vi "filter pipe - plot staff - more - V2.vi"(0 "omega  in":dbl[](array[numeric]), 1 "zin":cdb[](array[numeric]), 2 "z out":cdb[](array[numeric]), 3 "win omega":dbl[](array[numeric]), 4 "phase":dbl[](array[numeric]), 5 "dz/domega in":cdb[](array[numeric]), 6 "center":cdb, 7 "plots: filter related":T6, 8 "norm":dbl, 9 "parameters: complex fit":T1={"main VI path"=path "", "scale factor"=3.0, "# of grid points"=200, "parameters: wavepacket"={"R"=0.5, "wave number"=22.0, "delta k"=7.0, "radii vector"=[], "radial section"=[], "wave vector"=22.0, "wavepacket is"=TRUE}, "span"=0.27789, "interference ?"=enum."cp z center", "filter method"=enum."three"} {"span" min=0.0 max=0.5 step=1e-05 scale=0.0001..0.5 scale format="%#_5f"; "parameters: wavepacket"."delta k" format="%#_3f"; "parameters: wavepacket"."wave number" format="%#_3f"; "parameters: wavepacket"."R" format="%#_3f"}, 11 "tale of three indices -- int -- control":T7={"left"=0, "center"=0, "right"=0, "right most"=0, "left most"=0, "window"=0, "max win factor"=2, "max win"=2, "min win"=2}, 13 "lorentzian":T4={"Amplitude"=-1.0311345636926572, "omega(0)"=-1.0311345636926572, "Gamma"=-1.0311345636926572, "phase"=-1.0311345636926572, "Q"=-1.0311345636926572, "Norm  Ampl"=-1.0311345636926572, "z (inf)"=-1.0311345636926572+0.0i, "4corners"={"z (-pi/2)"=-1.0311345636926572+0.5736824521422934i, "z(inf)"=-0.5200164984937075+1.0975277942502903i, "z (pi/2)"=-1.0311345636926572+0.5736824521422934i, "z center"=-0.5136528600391839+0.580046090596817i, "z(0)"=-0.5200164984937075+1.0975277942502903i, "radius"=-1.0311345636926572}} {"z (inf)" format="%#9_9f"; "Q" format="%#9_9f"; "phase" format="%#9_9f"; "Gamma" format="%#9_9f"; "omega(0)" format="%#9_9f"}) -> ()   [LabVIEW 2015]
uses:
  tale of three indices -- int -- control.ctl
  plot refs -- filter related.ctl
  lorentzian.ctl
  circle corners.ctl
  peak -- parameters -- complex fit.ctl
  wavepacket.ctl
  filter method control.ctl
  four-corner circle transformation.ctl
  generate linear region.vi
panel:
  out "size(s)":i32
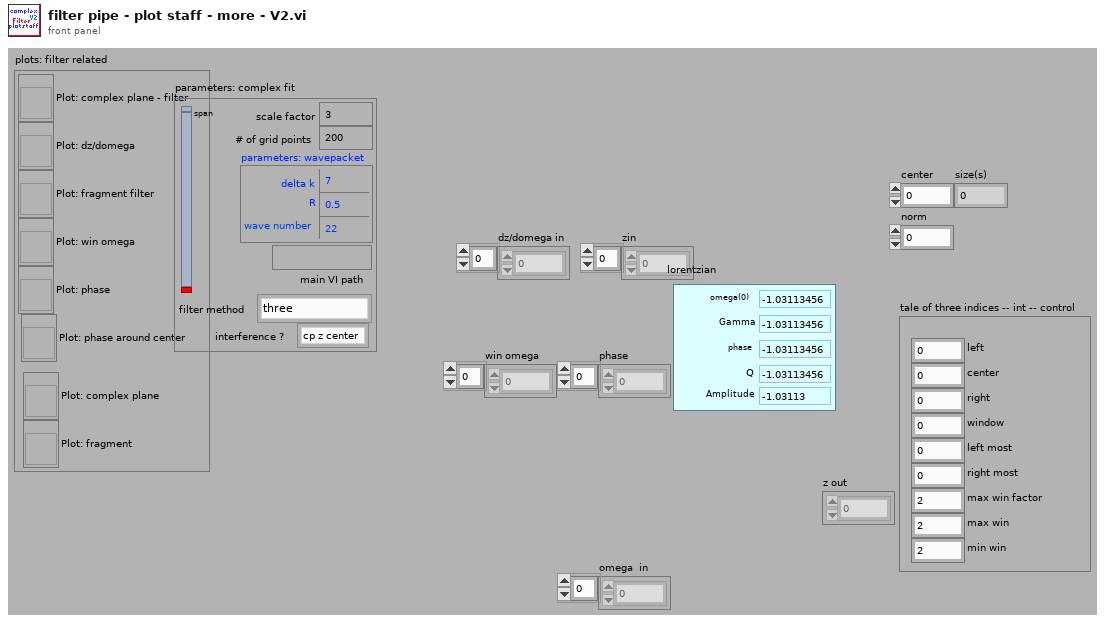
[diagram p1: front panel]
types:
  T1 = typedef "peak -- parameters -- complex fit.ctl" = cluster{"main VI path":path, "scale factor":dbl, "# of grid points":i32, "parameters: wavepacket":T2, "span":dbl, "interference ?":enum16{"cp z center", "pm zcenter", "fancy"}, "filter method":T3}
  T2 = typedef "wavepacket.ctl" = cluster{"R":dbl, "wave number":dbl, "delta k":dbl, "radii vector":dbl[], "radial section":cdb[], "wave vector":dbl, "wavepacket is":bool}
  T3 = typedef "filter method control.ctl" = enum16{"four", "five", "one", "two", "three", "zero", "minus one", "minus two"}
  T4 = typedef "lorentzian.ctl" = cluster{"Amplitude":dbl, "omega(0)":dbl, "Gamma":dbl, "phase":dbl, "Q":dbl, "Norm  Ampl":dbl, "z (inf)":cdb, "4corners":T5}
  T5 = typedef "circle corners.ctl" = cluster{"z (-pi/2)":cdb, "z(inf)":cdb, "z (pi/2)":cdb, "z center":cdb, "z(0)":cdb, "radius":dbl}
  T6 = typedef "plot refs -- filter related.ctl" = cluster{"Plot: complex plane - filter":refnum<vi>, "Plot: dz/domega":refnum<vi>, "Plot: fragment filter":refnum<vi>, "Plot: win omega":refnum<vi>, "Plot: phase":refnum<vi>, "Plot: phase around center":refnum<vi>, "Plot: complex plane":refnum<vi>, "Plot: fragment":refnum<vi>}
  T7 = typedef "tale of three indices -- int -- control.ctl" = cluster{"left":i32, "center":i32, "right":i32, "right most":i32, "left most":i32, "window":i32, "max win factor":i32, "max win":i32, "min win":i32}
  T8 = typedef "four-corner circle transformation.ctl" = enum16{"z(c) z(inf)", "z(c) z(zero)", "fix phase", "calculate lorentzian", "z(0) z(+-pi/2)", "shift to zcenter"}
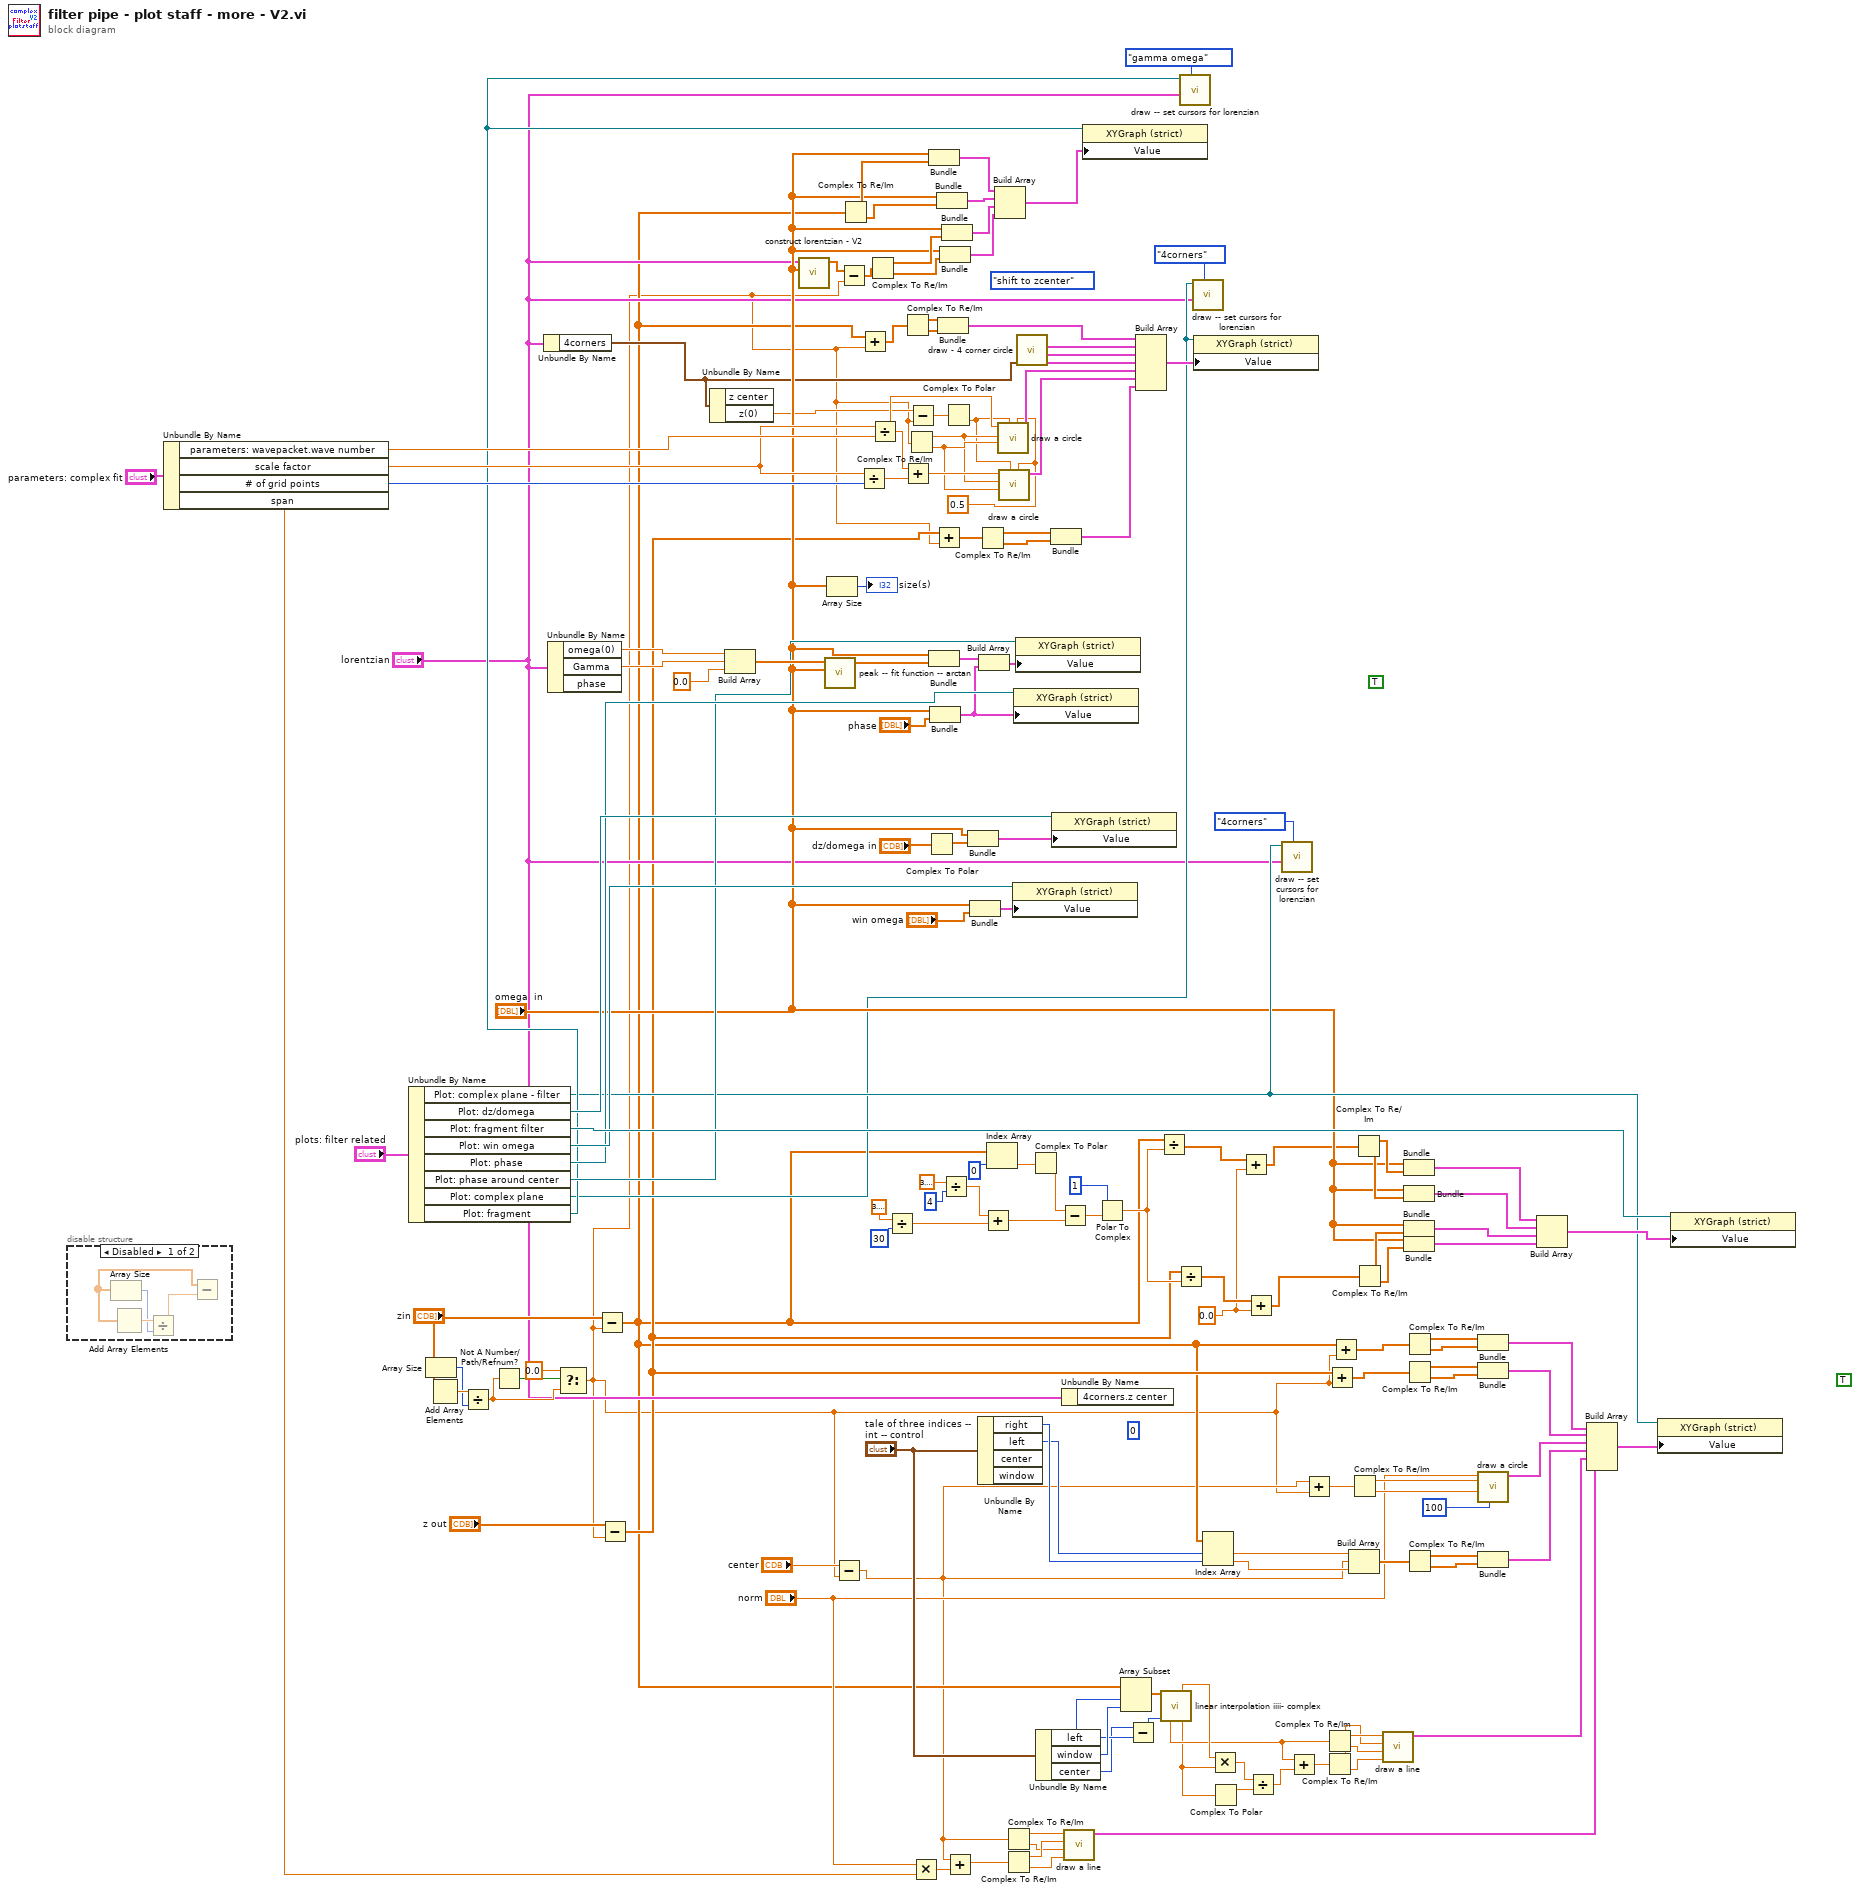
[diagram p0: block diagram]
diagram:
  w10 = 0.0 ("t")
  (unwired) four-corner_circle_transformation."shift to zcenter" ("4 corner circle transformation")
  (unwired) TRUE
  w58 = 0.5
  (unwired) 0
  (unwired) TRUE
  n1 = disable-structure shown="Disabled" {
    frame Disabled {
      n2 = Add Array Elements() -> (numeric array=w158:dbl[], sum=w160:dbl)
      n3 = Array Size(array=w158) -> (size(s)=w159:i32)
      n4 = Divide(x=w160, y=w159) -> (x/y=w157:dbl)
      n5 = Subtract(x=w158, y=w157) -> ()  [unwired: 1 out]
    }
    frame Enabled {
    }
  }
  n6 = Unbundle By Name("parameters: complex fit") -> ("parameters: wavepacket.wave number"=w56:dbl, "scale factor"=w51:dbl, "# of grid points"=w50:i32, "span"=w39:dbl)
  n7 = Unbundle By Name("plots: filter related") -> ("Plot: complex plane - filter"=w33:refnum<vi>, "Plot: dz/domega"=w81:refnum<vi>, "Plot: fragment filter"=w80:refnum<vi>, "Plot: win omega"=w79:refnum<vi>, "Plot: phase"=w73:refnum<vi>, "Plot: phase around center"=w71:refnum<vi>, "Plot: complex plane"=w28:refnum<vi>, "Plot: fragment"=w36:refnum<vi>)
  n8 = Array Size(array="zin") -> (size(s)=w17:i32)
  n9 = Add Array Elements(numeric array="zin") -> (sum=w18:cdb)
  n10 = Divide(x=w18, y=w17) -> (x/y=w16:cdb)
  n11 = Not A Number/Path/Refnum?(number/path/refnum=w16) -> (NaN/Path/Refnum?=w23:bool)
  n12 = Unbundle By Name("lorentzian") -> ("4corners"=w20:T5)
  n13 = Unbundle By Name("lorentzian") -> ("omega(0)"=w78:dbl, "Gamma"=w77:dbl)  [unwired: 1 out]
  n14 = Select(t=0.0, s=w23, f=w16) -> (s? t:f=w1:cdb)
  n15 = Subtract(x="zin", y=w1) -> (x-y=w5:cdb[])
  n16 = Subtract(x="z out", y=w1) -> (x-y=w7:cdb[])
  n17 = Unbundle By Name(w20) -> ("z(0)"=w25:cdb)  [unwired: 1 out]
  n18 = Build Array(w78, w77, 0.0 ("element")) -> (w76:dbl[])
  n19 = call "construct lorentzian - V2.vi"("omega  in"="omega  in", "lorentzian"="lorentzian") -> ("z out"=w27:cdb[])  [unwired: 9 in]
  n20 = call "peak -- fit function -- arctan.vi"("X"="omega  in", "a"=w76) -> ("f(X,a)"=w75:dbl[])  [unwired: 2 in, 2 out]
  n21 = Array Size(array="omega  in") -> (size(s)=→"size(s)":i32)
  n22 = Subtract(x="center", y=w1) -> (x-y=w3:cdb)
  n23 = Subtract(x=w27, y=w1) -> (x-y=w26:cdb[])
  n24 = Complex To Re/Im(x + iy=w5) -> (x=w47:dbl[], y=w48:dbl[])
  n25 = Divide(x=w51, y=w50) -> (x/y=w57:dbl)
  n26 = Add(x=w5, y=w1) -> (x+y=w4:cdb[])
  n27 = Complex To Re/Im(x + iy=w26) -> (x=w46:dbl[], y=w45:dbl[])
  n28 = Divide(x=w51, y=w56) -> (x/y=w65:dbl)
  n29 = Divide(x=3.141592653589793, y=30) -> (x/y=w89:dbl)
  n30 = Complex To Re/Im(x + iy=w4) -> (x=w68:dbl[], y=w67:dbl[])
  n31 = Add(x=w65, y=w57) -> (x+y=w64:dbl)
  n32 = Complex To Re/Im(x + iy=w1) -> (x=w61:dbl, y=w62:dbl)
  n33 = Subtract(x=w25, y=w1) -> (x-y=w60:cdb)
  n34 = Multiply(x="norm", y=w39) -> (x*y=w104:dbl)
  n35 = Complex To Polar(r * e^(i*theta)="dz/domega in") -> (r=w88:dbl[])  [unwired: 1 out]
  n36 = Bundle("omega  in"="omega  in", w47) -> (w44:cluster{"omega  in":dbl[], dbl[]})  [unwired: 1 in]
  n37 = Bundle("omega  in"="omega  in", "f(X,a)"=w75) -> (w74:cluster{"omega  in":dbl[], "f(X,a)":dbl[]})  [unwired: 1 in]
  n38 = Bundle("omega  in"="omega  in", "phase"="phase") -> (w72:cluster{"omega  in":dbl[], "phase":dbl[]})  [unwired: 1 in]
  n39 = Add(x=w7, y=w1) -> (x+y=w6:cdb[])
  n40 = Bundle("omega  in"="omega  in", w48) -> (w43:cluster{"omega  in":dbl[], dbl[]})  [unwired: 1 in]
  n41 = Bundle(w68, w67) -> (w69:cluster{dbl[], dbl[]})  [unwired: 1 in]
  n42 = Bundle("omega  in"="omega  in", w45) -> (w41:cluster{"omega  in":dbl[], dbl[]})  [unwired: 1 in]
  n43 = Divide(x=3.141592653589793, y=4) -> (x/y=w93:dbl)
  n44 = Bundle("omega  in"="omega  in", w46) -> (w42:cluster{"omega  in":dbl[], dbl[]})  [unwired: 1 in]
  n45 = Complex To Polar(r * e^(i*theta)=w60) -> (theta=w59:dbl)  [unwired: 1 out]
  n46 = Add(x=w3, y=w104) -> (x+y=w103:cdb)
  n47 = Bundle("omega  in"="omega  in", w88) -> (w86:cluster{"omega  in":dbl[], dbl[]})  [unwired: 1 in]
  n48 = Bundle("omega  in"="omega  in", "win omega"="win omega") -> (w84:cluster{"omega  in":dbl[], "win omega":dbl[]})  [unwired: 1 in]
  n49 = Complex To Re/Im(x + iy=w6) -> (x=w31:dbl[], y=w30:dbl[])
  n50 = Unbundle By Name("tale of three indices -- int -- control") -> ("right"=w131:i32, "left"=w128:i32)  [unwired: 2 out]
  n51 = Build Array(w74, w72) -> (w70:cluster{"omega  in":dbl[], "phase":dbl[]}[])
  n52 = Add(x=w93, y=w89) -> (x+y=w92:dbl)
  n53 = Index Array(array=w5, index=0) -> (element=w100:cdb)
  n54 = Build Array(w44, w43, w42, w41) -> (w40:cluster{"omega  in":dbl[], dbl[]}[])
  n55 = call "draw a circle.vi"("angular arc bounds"=w58, "angular arc center"=w59, "center Y"=w62, "center x"=w61, "radius"=w65) -> ("output cluster"=w66:cluster{dbl[], dbl[]})  [unwired: 6 in]
  n56 = call "draw a circle.vi"("angular arc bounds"=w58, "angular arc center"=w59, "center Y"=w62, "center x"=w61, "radius"=w64) -> ("output cluster"=w63:cluster{dbl[], dbl[]})  [unwired: 6 in]
  n57 = Complex To Re/Im(x + iy=w3) -> (x=w108:dbl, y=w105:dbl)
  n58 = Complex To Re/Im(x + iy=w103) -> (x=w106:dbl, y=w107:dbl)
  n59 = property class="XYGraph (strict)"(reference=w79, "Value"=w84) -> ()  [unwired: 1 in, 2 out]
  n60 = property class="XYGraph (strict)"(reference=w73, "Value"=w72) -> ()  [unwired: 1 in, 2 out]
  n61 = property class="XYGraph (strict)"(reference=w71, "Value"=w70) -> ()  [unwired: 1 in, 2 out]
  n62 = call "draw - 4 corner circle.vi"("4corners"=w20) -> ("line two"=w53:cluster{dbl[], dbl[]}, "line one"=w54:cluster{dbl[], dbl[]}, "circle"=w55:cluster{dbl[], dbl[]})  [unwired: 8 in]
  n63 = Complex To Polar(r * e^(i*theta)=w100) -> (theta=w96:dbl)  [unwired: 1 out]
  n64 = Unbundle By Name("tale of three indices -- int -- control") -> ("left"=w125:i32, "window"=w126:i32, "center"=w124:i32)
  n65 = Bundle(w31, w30) -> (w29:cluster{dbl[], dbl[]})  [unwired: 1 in]
  n66 = property class="XYGraph (strict)"(reference=w81, "Value"=w86) -> ()  [unwired: 1 in, 2 out]
  n67 = Subtract(x=w96, y=w92) -> (x-y=w95:dbl)
  n68 = Unbundle By Name("lorentzian") -> ()  [unwired: 1 out]
  n69 = call "draw a line.vi"("y1"=w107, "y0"=w105, "x1"=w106, "x0"=w108) -> ("output cluster"=w102:cluster{dbl[], dbl[]})  [unwired: 7 in]
  n70 = property class="XYGraph (strict)"(reference=w36, "Value"=w40) -> ()  [unwired: 1 in, 2 out]
  n71 = Polar To Complex(1:w95, 2:1) -> (0:w94:cdb)
  n72 = Array Subset(array=w5, index=w125, length=w126) -> (w127:cdb[])
  n73 = Subtract(x=w124, y=w125) -> (x-y=w123:i32)
  n74 = Build Array(w69, w55, w54, w53, w66, w63, w29) -> (w49:cluster{dbl[], dbl[]}[])
  n75 = Divide(x=w5, y=w94) -> (x/y=w12:cdb[])
  n76 = call "linear interpolation iiii- complex.vi"("Array"=w127, "center"=w123) -> ("directed sigma"=w120:dbl, "intercept"=w119:cdb, "slope"=w113:cdb)  [unwired: 5 in, 6 out]
  n77 = Divide(x=w7, y=w94) -> (x/y=w14:cdb[])
  n78 = call "draw -- set cursors for lorenzian.vi"("action"=enum16{"gamma omega", "4corners", "a"}."gamma omega", "lorentzian"="lorentzian", "Plot"=w36) -> ()  [unwired: 9 in]
  n79 = call "draw -- set cursors for lorenzian.vi"("action"=enum16{"gamma omega", "4corners", "a"}."4corners", "lorentzian"="lorentzian", "Plot"=w28) -> ()  [unwired: 9 in]
  n80 = property class="XYGraph (strict)"(reference=w28, "Value"=w49) -> ()  [unwired: 1 in, 2 out]
  n81 = Index Array(array=w5, index #1=w128, index #2=w131) -> (element #1=w133:cdb, element #2=w132:cdb)
  n82 = Multiply(x=w120, y=w113) -> (x*y=w111:cdb)
  n83 = Complex To Polar(r * e^(i*theta)=w113) -> (r=w112:dbl)  [unwired: 1 out]
  n84 = Add(x=w12, y=w10) -> (x+y=w11:cdb[])
  n85 = Add(x=w14, y=w10) -> (x+y=w13:cdb[])
  n86 = Divide(x=w111, y=w112) -> (x/y=w110:cdb)
  n87 = call "draw -- set cursors for lorenzian.vi"("action"=enum16{"gamma omega", "4corners", "a"}."4corners", "lorentzian"="lorentzian", "Plot"=w33) -> ()  [unwired: 9 in]
  n88 = Add(x=w119, y=w110) -> (x+y=w118:cdb)
  n89 = Add(x=w3, y=w1) -> (x+y=w2:cdb)
  n90 = Complex To Re/Im(x + iy=w119) -> (x=w121:dbl, y=w114:dbl)
  n91 = Complex To Re/Im(x + iy=w118) -> (x=w115:dbl, y=w117:dbl)
  n92 = Add(x=w7, y=w1) -> (x+y=w9:cdb[])
  n93 = Add(x=w5, y=w1) -> (x+y=w8:cdb[])
  n94 = Build Array(w133, w3, w132) -> (w130:cdb[])
  n95 = Complex To Re/Im(x + iy=w2) -> (x=w150:dbl, y=w149:dbl)
  n96 = Complex To Re/Im(x + iy=w11) -> (x=w140:dbl[], y=w139:dbl[])
  n97 = Complex To Re/Im(x + iy=w13) -> (x=w137:dbl[], y=w136:dbl[])
  n98 = call "draw a line.vi"("y1"=w117, "y0"=w114, "x1"=w115, "x0"=w121) -> ("output cluster"=w116:cluster{dbl[], dbl[]})  [unwired: 7 in]
  n99 = Bundle("omega  in"="omega  in", w140) -> (w138:cluster{"omega  in":dbl[], dbl[]})  [unwired: 1 in]
  n100 = Bundle("omega  in"="omega  in", w139) -> (w142:cluster{"omega  in":dbl[], dbl[]})  [unwired: 1 in]
  n101 = Bundle("omega  in"="omega  in", w137) -> (w135:cluster{"omega  in":dbl[], dbl[]})  [unwired: 1 in]
  n102 = Bundle("omega  in"="omega  in", w136) -> (w134:cluster{"omega  in":dbl[], dbl[]})  [unwired: 1 in]
  n103 = Complex To Re/Im(x + iy=w8) -> (x=w156:dbl[], y=w155:dbl[])
  n104 = Complex To Re/Im(x + iy=w9) -> (x=w154:dbl[], y=w153:dbl[])
  n105 = Complex To Re/Im(x + iy=w130) -> (x=w145:dbl[], y=w144:dbl[])
  n106 = Bundle(w156, w155) -> (w152:cluster{dbl[], dbl[]})  [unwired: 1 in]
  n107 = Bundle(w154, w153) -> (w151:cluster{dbl[], dbl[]})  [unwired: 1 in]
  n108 = call "draw a circle.vi"("number of points"=100, "center Y"=w149, "center x"=w150, "radius"="norm") -> ("output cluster"=w147:cluster{dbl[], dbl[]})  [unwired: 7 in]
  n109 = Bundle(w145, w144) -> (w143:cluster{dbl[], dbl[]})  [unwired: 1 in]
  n110 = Build Array(w138, w142, w135, w134) -> (w141:cluster{"omega  in":dbl[], dbl[]}[])
  n111 = Build Array(w152, w151, w147, w143, w116, w102) -> (w146:cluster{dbl[], dbl[]}[])
  n112 = property class="XYGraph (strict)"(reference=w33, "Value"=w146) -> ()  [unwired: 1 in, 2 out]
  n113 = property class="XYGraph (strict)"(reference=w80, "Value"=w141) -> ()  [unwired: 1 in, 2 out]
